vi "Process uService Go-NoGo Reply.vi"(8 "error in (no error)":errorcluster, 10 "Go-NoGo":T1, 11 "Tamer in":refnum<class "Tamer.lvclass">) -> (0 "error out":errorcluster, 3 "Tamer out":refnum<class "Tamer.lvclass">)   [LabVIEW 2020, in "Tamer.lvlib" / "Tamer.lvclass"]
uses:
  Tamer.lvclass
  TALOS/TALOS_PPL.lvlibp/Support VIs/Go-NoGo.ctl
  Reply.ctl
  Tamer.lvclass/Tamer.ctl
  TALOS/TALOS_PPL.lvlibp/Father of all uServices/Father of all uServices/Father of all uServices.lvclass
  TALOS/TALOS_PPL.lvlibp
  C:/Users/aegis/Documents/CIRCUS/TALOS/TALOS_PPL.lvlibp/Father of all uServices/Father of all uServices/Father of all uServices.lvclass
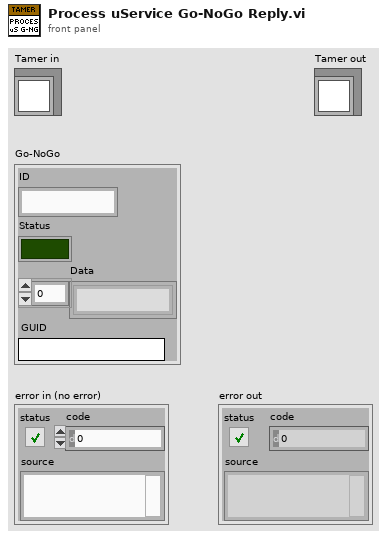
[diagram p1: front panel]
types:
  T1 = typedef "TALOS_PPL.lvlibp/Go-NoGo.ctl" = cluster{"ID":string, "Status":bool, "Data":string[], "GUID":string}
  T2 = typedef "Tamer.lvlib/Tamer.lvclass/Reply.ctl" = cluster{"ID":string, "Status":bool, "GUID":string}
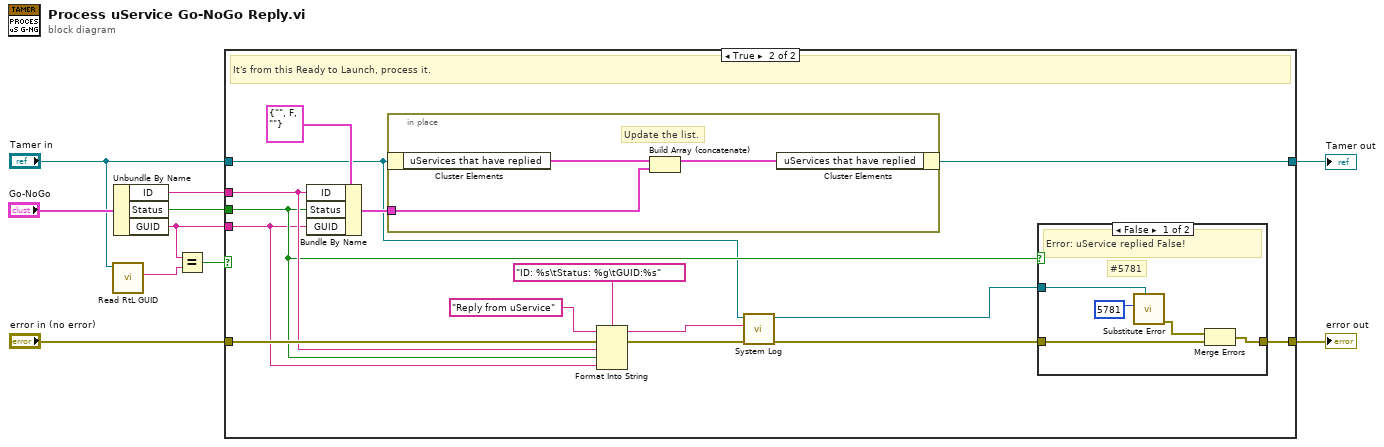
[diagram p0: block diagram]
diagram:
  n1 = call-dynamic "Read RtL GUID.vi"("Monkey in"="Tamer in") -> ("RtL GUID"=w2:string)  [unwired: 8 in, 2 out]
  n2 = Unbundle By Name("Go-NoGo") -> ("ID"=w6:string, "Status"=w5:bool, "GUID"=w3:string)
  n3 = Equal?(x=w3, y=w2) -> (x = y?=w1:bool)
  n4 = case shown="True" w1 {
    tunnel: "error in (no error)" -> [w11 w27]
    tunnel: [w11 w22] -> w9
    tunnel: [w12 w19] -> w8
    tunnel: w6 -> [_ w18]
    tunnel: w5 -> [_ w17]
    tunnel: "Tamer in" -> [w12 w16]
    tunnel: w3 -> [_ w15]
    frame False {
      # "It's from a previous Ready to Launch, disregard it."
    }
    frame True {
      # "It's from this Ready to Launch, process it."
      n5 = Bundle By Name(cluster=T2 {"ID"="", "Status"=FALSE, "GUID"=""} ("Reply"), "ID"=w18, "Status"=w17, "GUID"=w15) -> (w20:T2)
      n6 = in-place {
        in-place-border: w20 -> [w36]
        # "Update the list."
        n7 = in-place-cluster #1(w16) -> ("uServices that have replied"=w35:T2[])
        n8 = Build Array (concatenate)(w35, w36) -> (w34:T2[])
        n9 = in-place-cluster #1("uServices that have replied"=w34) -> (w19:refnum<class "Tamer.lvclass">)
      }
      n10 = Format Into String(format string="ID: %s\tStatus: %g\tGUID:%s", initial string="Reply from uService", error in=w27, w18, w17, w15) -> (resulting string=w25:string, error out=w24:errorcluster)
      n11 = call "System Log.vi"("error in (no error)"=w24, "Text to log"=w25, "uService Template in"=w16) -> ("error out"=w13:errorcluster, "uService Template out"=w14:refnum<class "Tamer.lvclass">)  [unwired: 7 in]
      n12 = case shown="False" w17 {
        tunnel: w13 -> [w32 w33]
        tunnel: [w31 w33] -> w22
        tunnel: w14 -> [w30 _]
        frame False {
          # "#5781"
          # "Error: uService replied False!"
          n13 = call "Substitute Error.vi"("LabVIEW Object"=w30, "Error Code"=5781) -> ("error out"=w28:errorcluster)  [unwired: 9 in]
          n14 = Merge Errors(w28, w32) -> (w31:errorcluster)
        }
        frame True {
          # "All OK"
        }
      }
    }
  }
  "error out" <- w9
  "Tamer out" <- w8
